vi "Coord vi Front and back camera.vi"(0 "Image Out":T10(plugin-control), 1 "Edge Options":T5={"Edge Polarity"=2, "Kernel Size"=5, "Width"=5, "Minimum Edge Strength"=50.0, "Interpolation Type"=enum."Bilinear Fixed", "Data Processing Method"=enum."Average"} {"Edge Polarity" items=["All Edges", "Rising Edges", "Falling Edges"]; "Minimum Edge Strength" format="%.2f"; "Width" step=2; "Kernel Size" step=2}, 2 "Search Direction":u32(ring)=2 items=["Left to Right", "Right to Left", "Top to Bottom", "Bottom to Top"], 3 "Line Options":T8={"Number of Lines"=1, "Type"=enum."First Edge Rake", "Min. Score"=10.0, "Max. Score"=1000.0, "Orientation"=0.0, "Angle Range"=10.0, "Angle Tolerance"=1.0, "Step Size"=10, "Min. SNR (db)"=0.0, "Min. Points (%)"=25.0, "Hough Iterations"=5} {"Min. Points (%)" min=0.0 max=100.0; "Min. SNR (db)" min=0.0; "Max. Score" min=0.0 max=1024.0; "Min. Score" min=0.0 max=1024.0 step=1.0}, 4 "Edge Options ROI 2":T5={"Edge Polarity"=0, "Kernel Size"=5, "Width"=5, "Minimum Edge Strength"=50.0, "Interpolation Type"=enum."Bilinear Fixed", "Data Processing Method"=enum."Average"} {"Edge Polarity" items=["All Edges", "Rising Edges", "Falling Edges"]; "Minimum Edge Strength" format="%.2f"; "Width" step=2; "Kernel Size" step=2}, 5 "Scan Direction ROI 2":u16(ring)=2 items=["Left To Right", "Right To Left", "Top To Bottom", "Bottom To Top"], 6 "Step Size ROI 2":u32=5, 7 "error in (no error)":errorcluster, 8 "ROI 1":T3 {"Contours"."Type" items=["No Selection", "Point", "Line", "Rectangle", "Oval", "Polygon", "Free", "Annulus", "Unused2", "Unused3", "Broken Line", "Free Hand Line", "Rotated Rectangle"]}, 9 "Process ROI 2":T4(ring)=enum."Get First + Last Edge", 10 "ROI 2":T3 {"Contours"."Type" items=["No Selection", "Point", "Line", "Rectangle", "Oval", "Polygon", "Free", "Annulus", "Unused2", "Unused3", "Broken Line", "Free Hand Line", "Rotated Rectangle"]}, 11 "Edge OptionsROI 3":T5={"Edge Polarity"=2, "Kernel Size"=5, "Width"=5, "Minimum Edge Strength"=50.0, "Interpolation Type"=enum."Bilinear Fixed", "Data Processing Method"=enum."Average"} {"Edge Polarity" items=["All Edges", "Rising Edges", "Falling Edges"]; "Minimum Edge Strength" format="%.2f"; "Width" step=2; "Kernel Size" step=2}, 12 "ROI 3":T2 {"Contours"."Type" items=["No Selection", "Point", "Line", "Rectangle", "Oval", "Polygon", "Freehand Region", "Annulus", "Unused2", "Unused3", "Broken Line", "Freehand Line", "Rotated Rectangle"]}, 13 "Search Direction ROI 3":u32(ring)=1 items=["Left to Right", "Right to Left", "Top to Bottom", "Bottom to Top"], 14 "OverlayOptions":T1, 15 "Line Options ROI 3":T8={"Number of Lines"=1, "Type"=enum."First Edge Rake", "Min. Score"=10.0, "Max. Score"=1000.0, "Orientation"=0.0, "Angle Range"=10.0, "Angle Tolerance"=1.0, "Step Size"=3, "Min. SNR (db)"=0.0, "Min. Points (%)"=25.0, "Hough Iterations"=5} {"Min. Points (%)" min=0.0 max=100.0; "Min. SNR (db)" min=0.0; "Max. Score" min=0.0 max=1024.0; "Min. Score" min=0.0 max=1024.0 step=1.0}) -> (20 "output cluster":T7, 27 "error out":errorcluster)   [LabVIEW 2019, in "Algorithm.lvclass"]
uses:
  FrameworkOverrides/Algorithm.lvclass
  <vilib>/vision/NI_Vision_Development_Module.lvlib
  <vilib>/vision/Measure.llb/Edge Polarity.ctl
  <vilib>/vision/Measure.llb/Edge Options.ctl
  <vilib>/vision/Measure.llb/Straight Edge Process.ctl
  <vilib>/vision/Measure.llb/Straight Edge Options.ctl
panel:
  out "Array":sgl[](array[numeric])
  out "Intersection Point":cluster{"X":sgl, "Y":sgl} {"Y" format="%.2f"; "X" format="%.2f"}
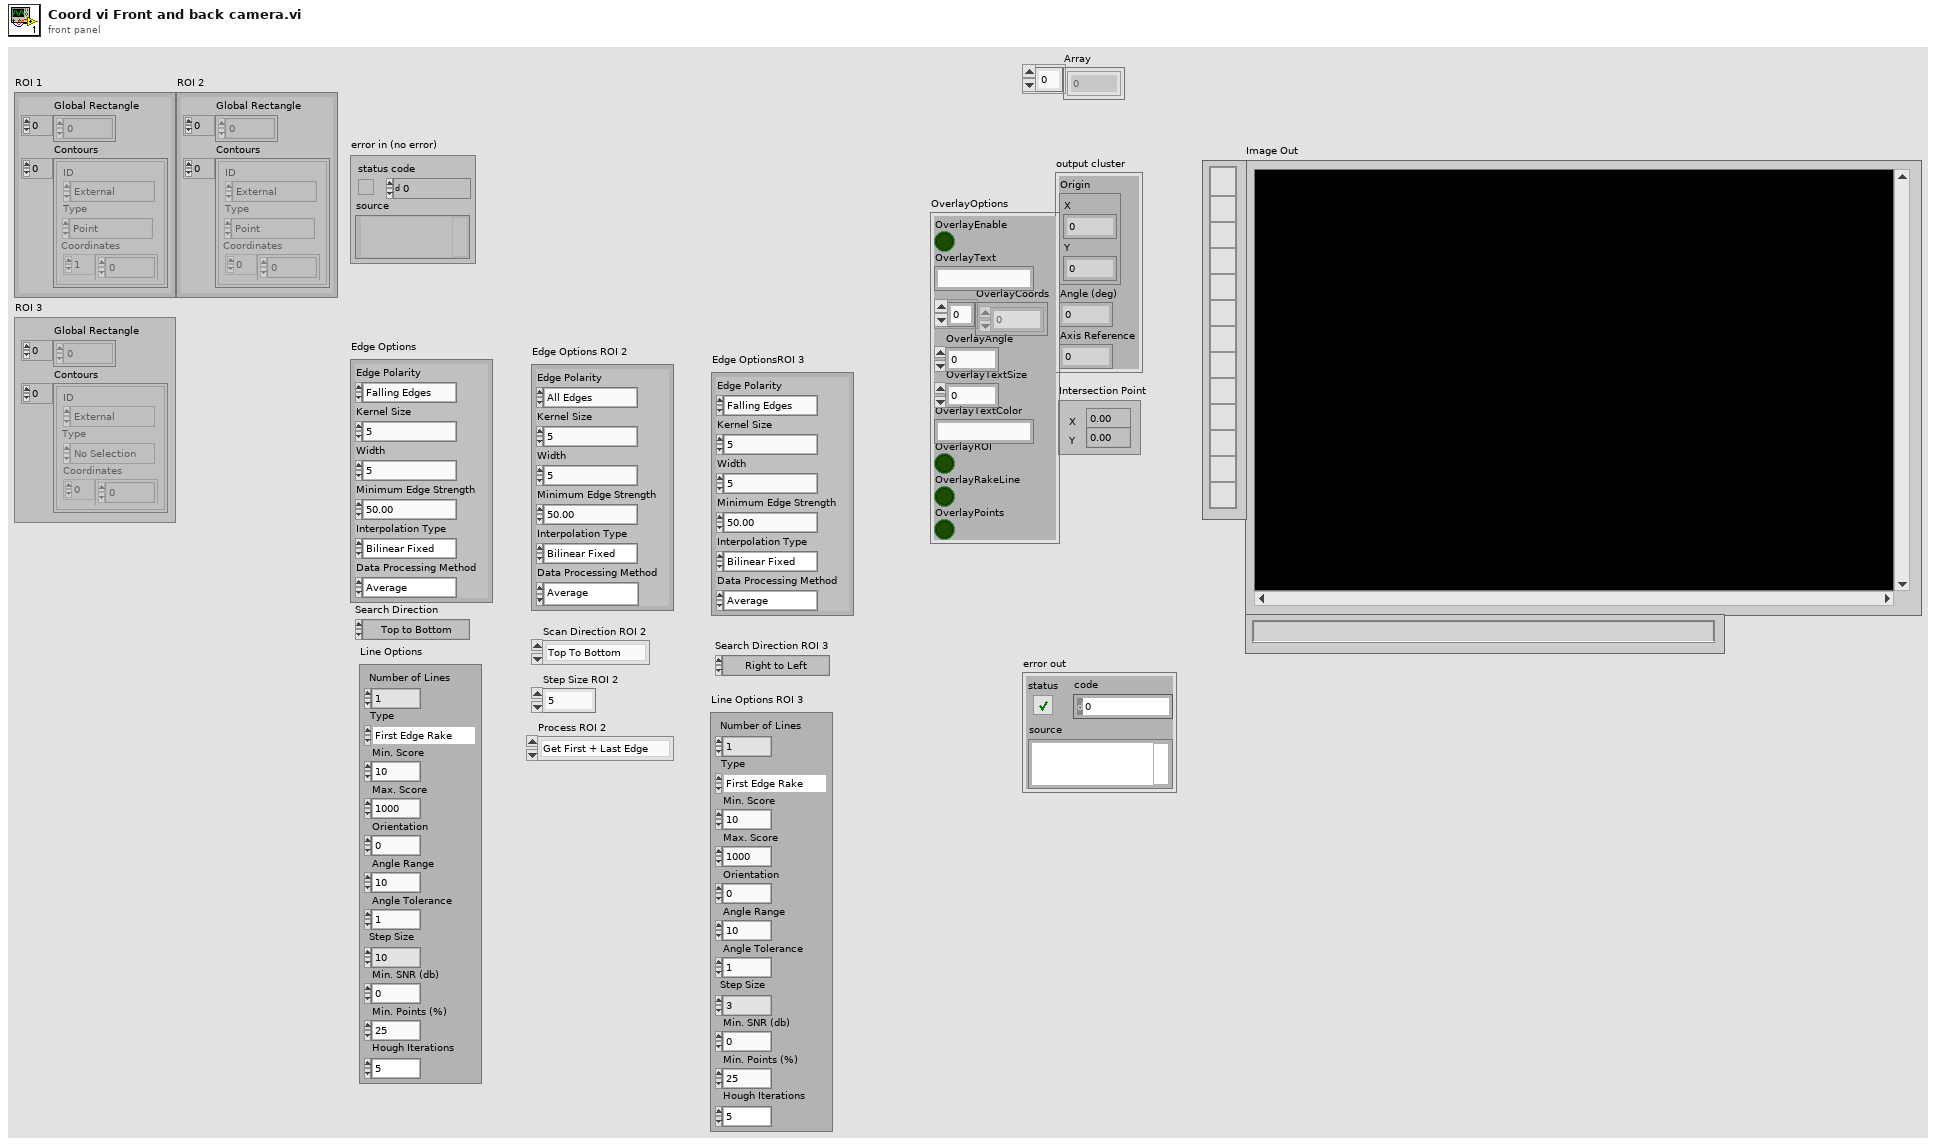
[diagram p1: front panel]
types:
  T1 = cluster{"OverlayEnable":bool, "OverlayText":string, "OverlayCoords":i32[], "OverlayAngle":i32, "OverlayTextSize":i32, "OverlayTextColor":string, "OverlayROI":bool, "OverlayRakeLine":bool, "OverlayPoints":bool}
  T2 = typedef "ROI Descriptor" = cluster{"Global Rectangle":i32[], "Contours":cluster{"ID":enum32{"External", "Internal"}, "Type":u32, "Coordinates":i32[]}[]}
  T3 = cluster{"Global Rectangle":i32[], "Contours":cluster{"ID":enum32{"External", "Internal"}, "Type":u32, "Coordinates":i32[]}[]}
  T4 = enum16{"Get First Edge", "Get First + Last Edge", "Get All Edges", "Get Best Edge"}
  T5 = typedef "Edge Options.ctl" = cluster{"Edge Polarity":T6, "Kernel Size":u32, "Width":u32, "Minimum Edge Strength":sgl, "Interpolation Type":enum32{"Zero Order", "Bilinear", "Quadratic", "Cubic", "Bilinear Fixed"}, "Data Processing Method":enum32{"Average", "Median"}}
  T6 = typedef "Edge Polarity.ctl" = u32
  T7 = cluster{"Origin":cluster{"X":sgl, "Y":sgl}, "Angle (deg)":sgl, "Axis Reference":u32}
  T8 = typedef "Straight Edge Options.ctl" = cluster{"Number of Lines":i32, "Type":T9, "Min. Score":dbl, "Max. Score":dbl, "Orientation":dbl, "Angle Range":dbl, "Angle Tolerance":dbl, "Step Size":u32, "Min. SNR (db)":dbl, "Min. Points (%)":dbl, "Hough Iterations":i32}
  T9 = typedef "Straight Edge Process.ctl" = enum32{"First Edge Rake", "Best Edge Rake", "Hough Edge Rake", "First Edge Projection", "Best Edge Projection"}
  T10 = typedef "IMAQ Image.ctl" = refnum<image>
  T11 = typedef "IMAQ Rectangle" = cluster{"Left":i32, "Top":i32, "Right":i32, "Bottom":i32, "Rotation":dbl}
  T12 = cluster{"Point 1":cluster{"X":sgl, "Y":sgl}, "Point 2":cluster{"X":sgl, "Y":sgl}}
  T13 = typedef "Edge New.ctl" = cluster{"Location (Pixel)":cluster{"X":sgl, "Y":sgl}, "Location (Real-World)":cluster{"X":sgl, "Y":sgl}, "Distance (Pixel)":dbl, "Distance (Real-World)":dbl, "Strength":dbl, "Noise":dbl, "Rising?":bool}
  T14 = typedef "Search Line.ctl" = cluster{"Start Point":cluster{"X":sgl, "Y":sgl}, "End Point":cluster{"X":sgl, "Y":sgl}, "Edge Info":T13[], "Edge Map":dbl[], "Calibration Valid":bool}
  T15 = cluster{"Point1 (Pixels)":cluster{"X":sgl, "Y":sgl}, "Point2 (Pixels)":cluster{"X":sgl, "Y":sgl}, "Point1 (Real-World)":cluster{"X":sgl, "Y":sgl}, "Point2 (Real-World)":cluster{"X":sgl, "Y":sgl}, "Angle (Pixel)":dbl, "Angle (Real-World)":dbl, "Score":dbl, "Straightness":dbl, "Average SNR (db)":dbl, "Calibration Valid":bool}[]
  T16 = cluster{"Point1 (Pixels)":cluster{"X":sgl, "Y":sgl}, "Point2 (Pixels)":cluster{"X":sgl, "Y":sgl}, "Point1 (Real-World)":cluster{"X":sgl, "Y":sgl}, "Point2 (Real-World)":cluster{"X":sgl, "Y":sgl}, "Angle (Pixel)":dbl, "Angle (Real-World)":dbl, "Score":dbl, "Straightness":dbl, "Average SNR (db)":dbl, "Calibration Valid":bool}
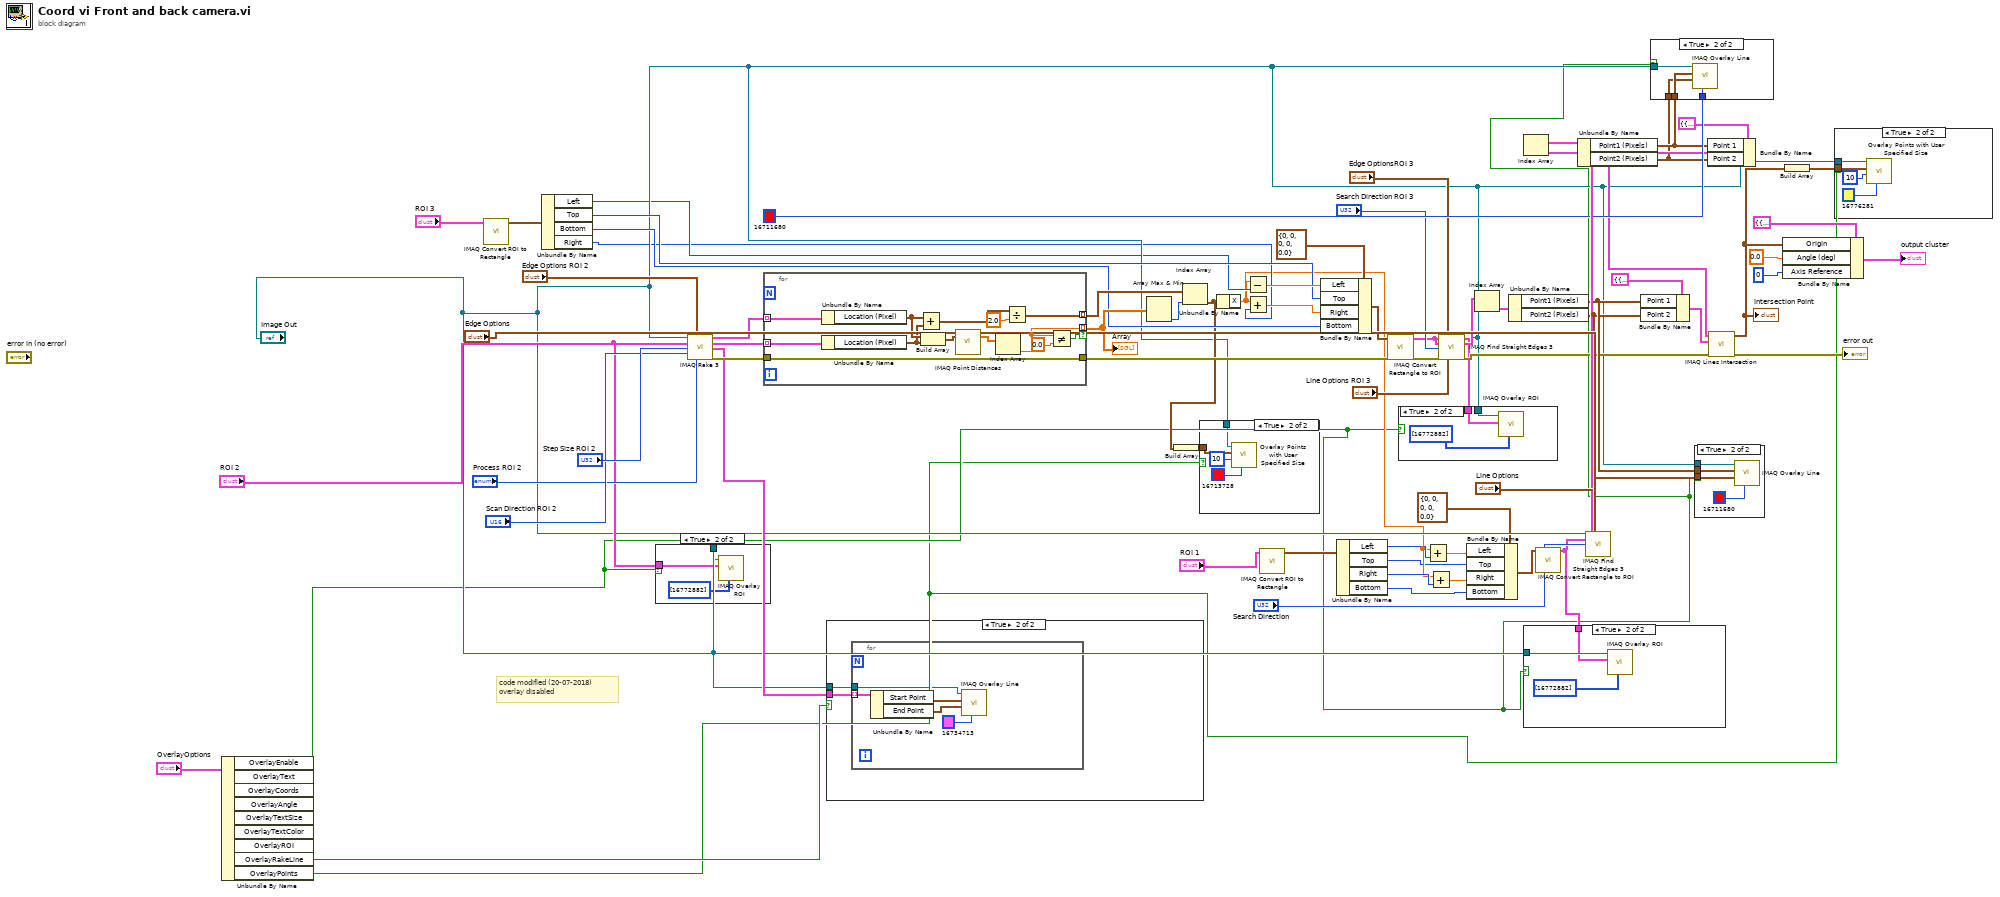
[diagram p0: block diagram]
diagram:
  # "code modified (20-07-2018)\noverlay disabled"
  n1 = Unbundle By Name("OverlayOptions") -> ("OverlayROI"=w2:bool, "OverlayRakeLine"=w3:bool, "OverlayPoints"=w1:bool)  [unwired: 6 out]
  n2 = call "IMAQ Convert ROI to Rectangle"("ROI Descriptor"="ROI 3") -> ("Rectangle"=w38:T11)  [unwired: 8 in, 1 out]
  n3 = Unbundle By Name(w38) -> ("Left"=w19:i32, "Top"=w33:i32, "Bottom"=w32:i32, "Right"=w18:i32)
  n4 = case shown="True" w2 {
    tunnel: "ROI 2" -> [_ w73]
    tunnel: "Image Out" -> [_ w72]
    frame False {
    }
    frame True {
      n5 = call "IMAQ Overlay ROI"("Colors (Green)"=u32[] [16772882], "ROI Descriptor"=w73, "Image"=w72) -> ()  [unwired: 7 in, 2 out]
    }
  }
  n6 = call "IMAQ Rake 3"("Image"="Image Out", "Edge Options"="Edge Options ROI 2", "ROI Descriptor"="ROI 2", "Step Size"="Step Size ROI 2", "Scan Direction"="Scan Direction ROI 2", "Process"="Process ROI 2") -> ("First Edges"=w43:T13[], "Last Edges"=w42:T13[], "Search Lines"=w24:T14[], "error out"=w37:errorcluster)  [unwired: 6 in]
  n7 = for {
    tunnel: w43 -> [w87] mode=indexing
    tunnel: w42 -> [w86] mode=indexing
    tunnel: [w82] -> w41 mode=indexing if=w81
    tunnel: [w76] -> w39 mode=indexing
    tunnel: w37 -> [w75]
    tunnel: [w75] -> w30
    n8 = Unbundle By Name(w87) -> ("Location (Pixel)"=w80:cluster{"X":sgl, "Y":sgl})
    n9 = Unbundle By Name(w86) -> ("Location (Pixel)"=w79:cluster{"X":sgl, "Y":sgl})
    n10 = Add(x=w80, y=w79) -> (x+y=w78:cluster{"X":sgl, "Y":sgl})
    n11 = Build Array(w80, w79) -> (w85:cluster{"X":sgl, "Y":sgl}[])
    n12 = call "IMAQ Point Distances"("Points"=w85) -> ("Distances"=w84:sgl[])  [unwired: 4 in, 1 out]
    n13 = Index Array(array=w84) -> (element=w82:sgl)  [unwired: 1 in]
    n14 = Divide(x=w78, y=sgl 2.0) -> (x/y=w76:cluster{"X":sgl, "Y":sgl})
    n15 = Not Equal?(x=w82, y=sgl 0.0) -> (x != y?=w81:bool)
  }
  "Array" <- w41
  n16 = case shown="True" w3 {
    tunnel: w24 -> [_ w89]
    tunnel: "Image Out" -> [_ w88]
    frame False {
    }
    frame True {
      n17 = for {
        tunnel: w89 -> [w94] mode=indexing
        tunnel: w88 -> [w91]
        n18 = Unbundle By Name(w94) -> ("Start Point"=w93:cluster{"X":sgl, "Y":sgl}, "End Point"=w92:cluster{"X":sgl, "Y":sgl})
        n19 = call "IMAQ Overlay Line"("Color"=u32 16734713, "End Point"=w92, "Start Point"=w93, "Image"=w91) -> ()  [unwired: 6 in, 2 out]
      }
    }
  }
  n20 = Array Max & Min(array=w41) -> (min index (indices)=w40:i32)  [unwired: 3 out]
  n21 = Index Array(array=w39, index=w40) -> (element=w28:cluster{"X":sgl, "Y":sgl})
  n22 = Build Array(w28) -> (w27:cluster{"X":sgl, "Y":sgl}[])
  n23 = case shown="True" w1 {
    tunnel: w27 -> [_ w98]
    tunnel: "Image Out" -> [_ w95]
    frame False {
    }
    frame True {
      n24 = call "Overlay Points with User Specified Size.vi"("Color"=u32 16713728, "Point Diameter (5)"=u32 10, "Points"=w98, "Image In"=w95) -> ()  [unwired: 6 in, 2 out]
    }
  }
  n25 = Unbundle By Name(w28) -> ("X"=w12:sgl)
  n26 = Subtract(x=w12, y=w19) -> (x-y=w35:sgl)
  n27 = Add(x=w12, y=w18) -> (x+y=w34:sgl)
  n28 = call "IMAQ Convert ROI to Rectangle"("ROI Descriptor"="ROI 1") -> ("Rectangle"=w15:T11)  [unwired: 8 in, 1 out]
  n29 = Bundle By Name(cluster=T11 {"Left"=0, "Top"=0, "Right"=0, "Bottom"=0, "Rotation"=0.0} ("Rectangle"), "Left"=w35, "Top"=w33, "Right"=w34, "Bottom"=w32) -> (w31:T11)
  n30 = Unbundle By Name(w15) -> ("Left"=w14:i32, "Top"=w9:i32, "Right"=w13:i32, "Bottom"=w7:i32)
  n31 = call "IMAQ Convert Rectangle to ROI"("error in (no error)"=w30, "Rectangle"=w31) -> ("error out"=w29:errorcluster, "ROI Descriptor"=w25:T2)  [unwired: 7 in]
  n32 = case shown="True" w2 {
    tunnel: w25 -> [_ w101]
    tunnel: "Image Out" -> [_ w99]
    frame False {
    }
    frame True {
      n33 = call "IMAQ Overlay ROI"("Colors (Green)"=u32[] [16772882], "ROI Descriptor"=w101, "Image"=w99) -> ()  [unwired: 7 in, 2 out]
    }
  }
  n34 = Add(x=w12, y=w14) -> (x+y=w10:sgl)
  n35 = Add(x=w12, y=w13) -> (x+y=w8:sgl)
  n36 = call "IMAQ Find Straight Edges 3"("Image"="Image Out", "Edge Options"="Edge OptionsROI 3", "ROI Descriptor"=w25, "Search Direction"="Search Direction ROI 3", "error in (no error)"=w29, "Line Options"="Line Options ROI 3") -> ("Straight Edges"=w62:T15, "error out"=w26:errorcluster)  [unwired: 5 in, 3 out]
  n37 = Bundle By Name(cluster=T11 {"Left"=0, "Top"=0, "Right"=0, "Bottom"=0, "Rotation"=0.0} ("Rectangle"), "Left"=w10, "Top"=w9, "Right"=w8, "Bottom"=w7) -> (w6:T11)
  n38 = Index Array(array=w62) -> (element=w63:T16)  [unwired: 1 in]
  n39 = Unbundle By Name(w63) -> ("Point1 (Pixels)"=w55:cluster{"X":sgl, "Y":sgl}, "Point2 (Pixels)"=w54:cluster{"X":sgl, "Y":sgl})
  n40 = call "IMAQ Convert Rectangle to ROI"("Rectangle"=w6) -> ("ROI Descriptor"=w5:T2)  [unwired: 8 in, 1 out]
  n41 = case shown="True" w2 {
    tunnel: "Image Out" -> [_ w103]
    tunnel: w5 -> [_ w102]
    frame False {
    }
    frame True {
      n42 = call "IMAQ Overlay ROI"("Colors (Green)"=u32[] [16772882], "ROI Descriptor"=w102, "Image"=w103) -> ()  [unwired: 7 in, 2 out]
    }
  }
  n43 = call "IMAQ Find Straight Edges 3"("Image"="Image Out", "Edge Options"="Edge Options", "ROI Descriptor"=w5, "Search Direction"="Search Direction", "Line Options"="Line Options") -> ("Straight Edges"=w69:T15)  [unwired: 6 in, 4 out]
  n44 = Index Array(array=w69) -> (element=w68:T16)  [unwired: 1 in]
  n45 = Unbundle By Name(w68) -> ("Point1 (Pixels)"=w57:cluster{"X":sgl, "Y":sgl}, "Point2 (Pixels)"=w56:cluster{"X":sgl, "Y":sgl})
  n46 = Bundle By Name(cluster=T12 {"Point 1"={"X"=0.0, "Y"=0.0}, "Point 2"={"X"=0.0, "Y"=0.0}} ("Line 1"), "Point 1"=w55, "Point 2"=w54) -> (w58:T12)
  n47 = case shown="True" w2 {
    tunnel: u32 16711680 ("Color") -> [_ w108]
    tunnel: w57 -> [_ w107]
    tunnel: w56 -> [_ w106]
    tunnel: "Image Out" -> [_ w105]
    frame False {
    }
    frame True {
      n48 = call "IMAQ Overlay Line"("Color"=w108, "End Point"=w106, "Start Point"=w107, "Image"=w105) -> ()  [unwired: 6 in, 2 out]
    }
  }
  n49 = case shown="True" w2 {
    tunnel: w55 -> [_ w111]
    tunnel: w54 -> [_ w110]
    tunnel: "Image Out" -> [_ w109]
    frame False {
    }
    frame True {
      n50 = call "IMAQ Overlay Line"("Color"=u32 16711680, "End Point"=w110, "Start Point"=w111, "Image"=w109) -> ()  [unwired: 6 in, 2 out]
    }
  }
  n51 = Bundle By Name(cluster=T12 {"Point 1"={"X"=0.0, "Y"=0.0}, "Point 2"={"X"=0.0, "Y"=0.0}} ("Line 1"), "Point 1"=w57, "Point 2"=w56) -> (w59:T12)
  n52 = call "IMAQ Lines Intersection"("error in (no error)"=w26, "Line 2"=w58, "Line 1"=w59) -> ("error out"=→"error out":errorcluster, "Intersection Point"=w49:cluster{"X":sgl, "Y":sgl})  [unwired: 6 in, 1 out]
  "Intersection Point" <- w49
  n53 = Bundle By Name(cluster=T7 {"Origin"={"X"=0.0, "Y"=0.0}, "Angle (deg)"=0.0, "Axis Reference"=0} ("Coordinate System"), "Origin"=w49, "Angle (deg)"=sgl 0.0, "Axis Reference"=u32 0) -> (→"output cluster":T7)
  n54 = Build Array(w49) -> (w53:cluster{"X":sgl, "Y":sgl}[])
  n55 = case shown="True" w1 {
    tunnel: w53 -> [_ w116]
    tunnel: "Image Out" -> [_ w113]
    frame False {
    }
    frame True {
      n56 = call "Overlay Points with User Specified Size.vi"("Color"=u32 16776281, "Point Diameter (5)"=u32 10, "Points"=w116, "Image In"=w113) -> ()  [unwired: 6 in, 2 out]
    }
  }
